vi "P2.vi"() -> ()   [LabVIEW 2018]
uses:
  <vilib>/imath/engines/lvmath2/RunTimeEngine/ErrorHandling/NIMS_Finalize Error.vi
  <vilib>/imath/engines/lvmath2/RunTimeEngine/NodeEndStatement/NIMS_NodeEndStatement_Output.vi
  <vilib>/imathl/engines/lvmath/Functions/Error Handling/Create Error.vi
  <vilib>/imath/engines/lvmath2/RunTimeEngine/ErrorHandling/NIMS_Create Error From Enums.vi
  <vilib>/imath/engines/lvmath2/RunTimeEngine/BuiltInFunctions/plot/NIMS_plot(G, Str).vi
  <vilib>/imath/engines/lvmath2/RunTimeEngine/BuiltInFunctions/fir_win/NIMS_fir_win(I32,V,V,Str).vi
  <vilib>/imath/engines/lvmath2/RunTimeEngine/BuiltInFunctions/figure/NIMS_figure(I32).vi
  <vilib>/imath/engines/lvmath2/RunTimeEngine/BuiltInFunctions/freqzd/NIMS_NoOutput_freqzd().vi
  <vilib>/imath/engines/lvmath2/RunTimeEngine/BuiltInFunctions/fir_win/NIMS_fir_win(I32,V,Str,V,Str).vi
  <vilib>/imath/engines/lvmath2/RunTimeEngine/BuiltInFunctions/win_hann2/NIMS_win_hann2.vi
  <vilib>/imath/engines/lvmath2/RunTimeEngine/BuiltInFunctions/win_bartlett/NIMS_win_bartlett.vi
  <vilib>/imath/engines/lvmath2/RunTimeEngine/BuiltInFunctions/win_cheby/NIMS_win_cheby.vi
  <vilib>/imath/engines/lvmath2/RunTimeEngine/BuiltInFunctions/win_blackman/NIMS_win_blackman.vi
panel:
  in  "fs":dbl
  in  "wn":dbl
  out "Arreglo":dbl[](array[numeric])
  in  "n":dbl
  in  "?":bool
  in  "1":bool
  in  "Ch":bool
  in  "H":bool
  in  "BM":bool
  in  "B":bool
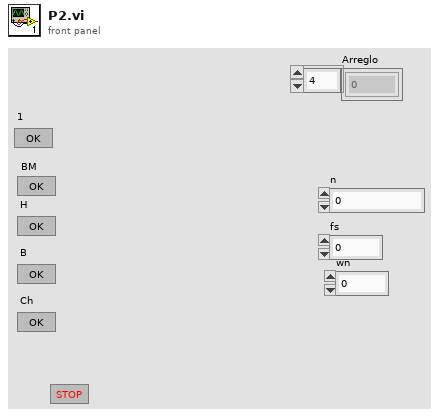
[diagram p1: front panel]
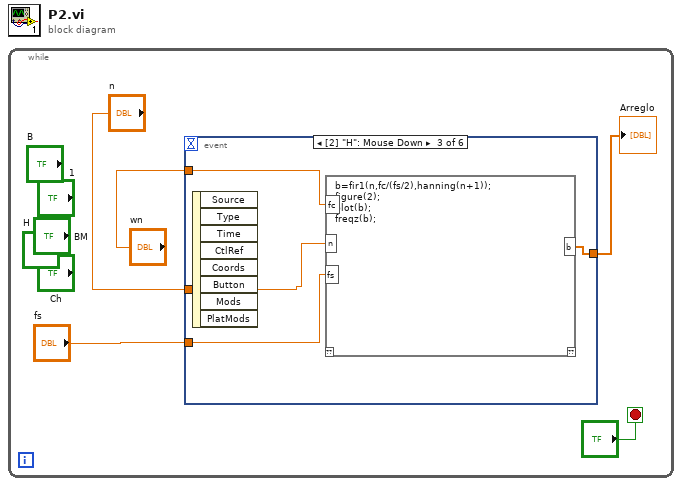
[diagram p0: block diagram]
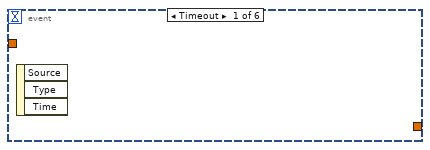
[diagram p2: hidden frame]
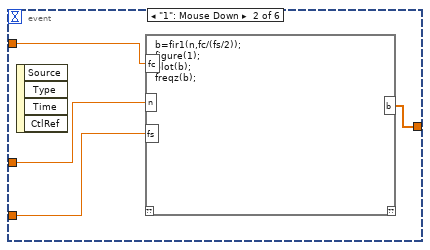
[diagram p3: hidden frame]
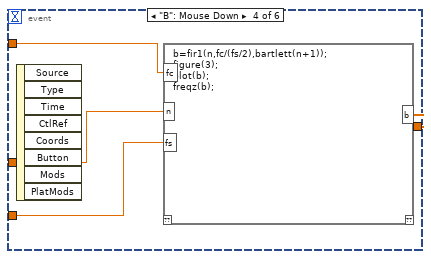
[diagram p4: hidden frame]
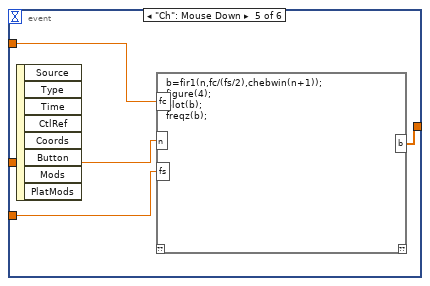
[diagram p5: hidden frame]
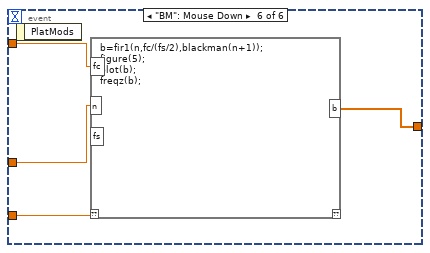
[diagram p6: hidden frame]
diagram:
  n1 = while {
    stop <- "?" stop-if-true
    n2 = event shown="[2] \"H\": Mouse Down" {
      selector: _ -> [_ _ _ _ _ _]
      dyn-events: _ -> [_ _ _ _ _ _]
      timeout: _ -> [_ _ _ _ _ _]
      tunnel: "n" -> [_ w7 w105 w209 w316 w421]
      tunnel: [_ w9 w107 w212 w314 w420] -> w3
      tunnel: "wn" -> [_ w8 w106 w211 w317 w422]
      tunnel: "fs" -> [_ w6 w104 w210 w315 w419]
      event Timeout {
        n3 = event-data() -> ()  [unwired: 1 in, 3 out]
      }
      event "1": Mouse Down {
        n4 = event-data() -> ()  [unwired: 1 in, 4 out]
        n5 = mathscript code="b=fir1(n,fc/(fs/2));\nfigure(1);\nplot(b);\nfreqz(b);"("n"=w7, "fc"=w8, "fs"=w6) -> ("b"=w9:dbl[])  [unwired: 1 in, 1 out]
      }
      event "H": Mouse Down {
        n6 = event-data() -> ()  [unwired: 1 in, 8 out]
        n7 = mathscript code="b=fir1(n,fc/(fs/2),hanning(n+1));\nfigure(2);\nplot(b);\nfreqz(b);"("n"=w105, "fc"=w106, "fs"=w104) -> ("b"=w107:dbl[])  [unwired: 1 in, 1 out]
      }
      event "B": Mouse Down {
        n8 = event-data() -> ()  [unwired: 1 in, 8 out]
        n9 = mathscript code="b=fir1(n,fc/(fs/2),bartlett(n+1));\nfigure(3);\nplot(b);\nfreqz(b);"("n"=w209, "fc"=w211, "fs"=w210) -> ("b"=w212:dbl[])  [unwired: 1 in, 1 out]
      }
      event "Ch": Mouse Down {
        n10 = event-data() -> ()  [unwired: 1 in, 8 out]
        n11 = mathscript code="b=fir1(n,fc/(fs/2),chebwin(n+1));\nfigure(4);\nplot(b);\nfreqz(b);"("n"=w316, "fc"=w317, "fs"=w315) -> ("b"=w314:dbl[])  [unwired: 1 in, 1 out]
      }
      event "BM": Mouse Down {
        n12 = event-data() -> ()  [unwired: 1 in, 1 out]
        n13 = mathscript code="b=fir1(n,fc/(fs/2),blackman(n+1));\nfigure(5);\nplot(b);\nfreqz(b);"("n"=w421, "fc"=w422, "fs"=w419) -> ("b"=w420:dbl[])  [unwired: 1 in, 1 out]
      }
    }
    "Arreglo" <- w3
  }
